vi "Driver Filename to IDs.vi"(5 "Driver Filename (\"\")":string) -> (0 "Extension":string, 1 "sType":string, 2 "sxDriverId":string)   [LabVIEW 2011]
uses:
  Summitek EXT/OpenG EXT/file/file.llb/Strip Path Extension - String__ogtk.vi
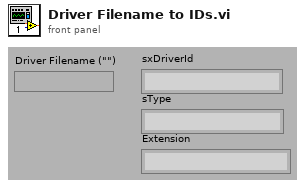
[diagram p1: front panel]
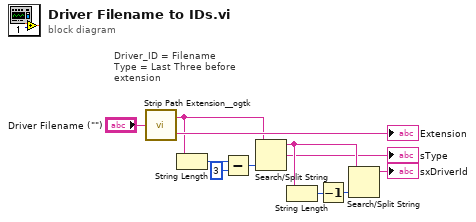
[diagram p0: block diagram]
diagram:
  # "Driver_ID = Filename\nType = Last Three before\nextension"
  n1 = call-poly "Strip Path Extension__ogtk.vi"("path"="Driver Filename (\"\")") -> ("root"=w1:string, "extension"=→"Extension":string)
  n2 = String Length(string=w1) -> (length=w11:i32)
  n3 = Subtract(x=w11, y=3) -> (x-y=w9:i32)
  n4 = Search/Split String(string=w1, offset (0)=w9) -> (substring before match=w7:string, match + rest of string=→"sType":string)  [unwired: 2 out]
  n5 = String Length(string=w7) -> (length=w8:i32)
  n6 = Decrement(x=w8) -> (x-1=w6:i32)
  n7 = Search/Split String(string=w7, offset (0)=w6) -> (substring before match=→"sxDriverId":string)  [unwired: 3 out]
